vi "control_chart_axis.vi"(8 "stop":refnum<vi>, 9 "chart_array":refnum<vi>[](array[refnum]), 10 "chart_2":refnum<vi>, 11 "chart_1":refnum<vi>) -> ()   [LabVIEW 2019]
panel:
  in  "range_p1h":bool
  in  "range_p10m":bool
  in  "range_p5m":bool
  in  "chart_x_range":u32 caption="Time range"
  in  "auto_x_scale":bool caption="Time Scale"
  in  "auto_y_scale":bool caption="Vertical Scale"
  # "min"
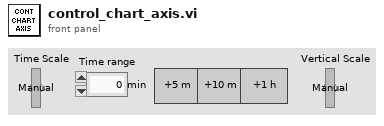
[diagram p1: front panel]
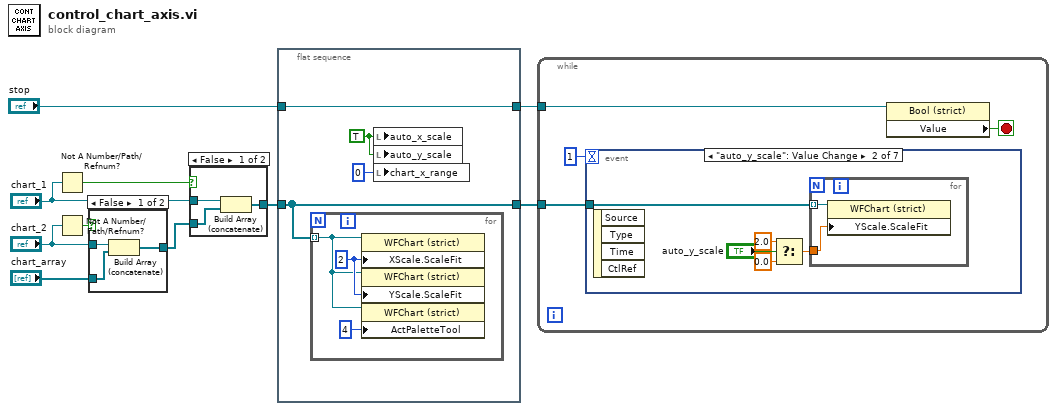
[diagram p0: block diagram]
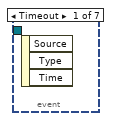
[diagram p4: hidden frame]
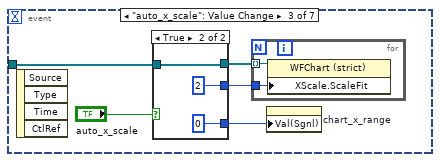
[diagram p5: hidden frame]
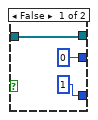
[diagram p6: hidden frame]
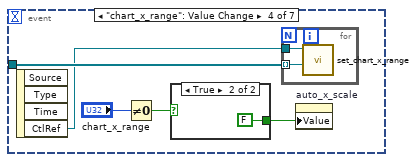
[diagram p7: hidden frame]
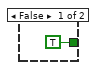
[diagram p8: hidden frame]
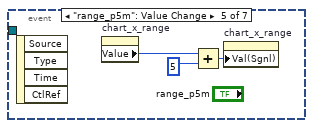
[diagram p9: hidden frame]
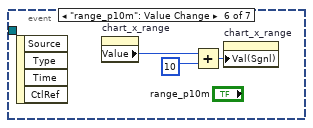
[diagram p10: hidden frame]
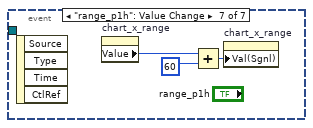
[diagram p11: hidden frame]
diagram:
  n1 = Not A Number/Path/Refnum?(number/path/refnum="chart_1") -> (NaN/Path/Refnum?=w7:bool)
  n2 = Not A Number/Path/Refnum?(number/path/refnum="chart_2") -> (NaN/Path/Refnum?=w4:bool)
  n3 = case shown="False" w4 {
    tunnel: "chart_array" -> [w12 w14]
    tunnel: "chart_2" -> [w13 _]
    tunnel: [w11 w14] -> w1
    frame False {
      n4 = Build Array (concatenate)(w13, w12) -> (w11:refnum<vi>[])
    }
    frame True {
    }
  }
  n5 = case shown="False" w7 {
    tunnel: "chart_1" -> [w16 _]
    tunnel: [w17 w18] -> w5
    tunnel: w1 -> [w15 w18]
    frame False {
      n6 = Build Array (concatenate)(w16, w15) -> (w17:refnum<vi>[])
    }
    frame True {
    }
  }
  n7 = flat-sequence {
    tunnel: w5 -> [w20]
    tunnel: [w20] -> w10
    tunnel: [w19] -> w9
    tunnel: "stop" -> [w19]
    frame #0 {
      w21 = TRUE ("auto_x_scale")
      n8 = for {
        tunnel: w20 -> [w24] mode=indexing
        w25 = u8 2 ("X Scale.Scale Fit")
        n9 = property class="WFChart (strict)"(reference=w24, "XScale.ScaleFit"=w25) -> ()  [unwired: 1 in, 2 out]
        n10 = property class="WFChart (strict)"(reference=w24, "YScale.ScaleFit"=w25) -> ()  [unwired: 1 in, 2 out]
        n11 = property class="WFChart (strict)"(reference=w24, "ActPaletteTool"=4 ("Palette:Active Tool")) -> ()  [unwired: 1 in, 2 out]
      }
      n12 = local write "auto_x_scale"(w21) -> ()
      n13 = local write "auto_y_scale"(w21) -> ()
      n14 = local write "chart_x_range"(u32 0 ("chart_x_range")) -> ()
    }
  }
  n15 = while {
    tunnel: w10 -> [w28]
    tunnel: w9 -> [w26]
    stop <- w27 stop-if-true
    n16 = event shown="[1] \"auto_y_scale\": Value Change" {
      selector: _ -> [_ _ _ _ _ _ _]
      dyn-events: _ -> [_ _ _ _ _ _ _]
      timeout: 1 -> [_ _ _ _ _ _ _]
      tunnel: w28 -> [_ w30 w38 w51 _ _ _]
      event Timeout {
        n17 = event-data() -> ()  [unwired: 1 in, 3 out]
      }
      event "auto_y_scale": Value Change {
        n18 = event-data() -> ()  [unwired: 1 in, 4 out]
        n19 = Select(t=2.0, s="auto_y_scale", f=0.0) -> (s? t:f=w33:dbl)
        n20 = for {
          tunnel: w33 -> [w36]
          tunnel: w30 -> [w35] mode=indexing
          n21 = property class="WFChart (strict)"(reference=w35, "YScale.ScaleFit"=w36) -> ()  [unwired: 1 in, 2 out]
        }
      }
      event "auto_x_scale": Value Change {
        n22 = event-data() -> ()  [unwired: 1 in, 4 out]
        n23 = case shown="True" "auto_x_scale" {
          tunnel: [1 ("chart_x_range") 0 ("chart_x_range")] -> w40
          tunnel: [u8 0 ("X Scale.Scale Fit") u8 2 ("X Scale.Scale Fit")] -> w39
          tunnel: w38 -> [w44 w47]
          tunnel: [w44 w47] -> w37
          frame False {
          }
          frame True {
          }
        }
        n24 = for {
          tunnel: w39 -> [w43]
          tunnel: w37 -> [w42] mode=indexing
          n25 = property class="WFChart (strict)"(reference=w42, "XScale.ScaleFit"=w43) -> ()  [unwired: 1 in, 2 out]
        }
        n26 = property on="chart_x_range" class="DigNum (strict)"("Val(Sgnl)"=w40) -> ()  [unwired: 2 in, 2 out]
      }
      event "chart_x_range": Value Change {
        n27 = event-data() -> ("CtlRef"=w50:refnum<vi>)  [unwired: 1 in, 3 out]
        n28 = Not Equal To 0?(x="chart_x_range") -> (x != 0?=w53:bool)
        n29 = case shown="True" w53 {
          tunnel: [TRUE ("auto_x_scale") FALSE ("auto_x_scale")] -> w52
          frame False {
          }
          frame True {
          }
        }
        n30 = for {
          tunnel: w51 -> [w56] mode=indexing
          tunnel: w50 -> [w55]
          n31 = call "set_chart_x_range.vi"("ref_chart"=w56, "ref_x_range"=w55) -> ()  [unwired: 10 in]
        }
        n32 = property on="auto_x_scale" class="Bool (strict)"("Value"=w52) -> ()  [unwired: 2 in, 2 out]
      }
      event "range_p5m": Value Change {
        n33 = event-data() -> ()  [unwired: 1 in, 4 out]
        n34 = property on="chart_x_range" class="DigNum (strict)"() -> ("Value"=w61:u32)  [unwired: 2 in, 2 out]
        n35 = Add(x=w61, y=5) -> (x+y=w60:u32)
        n36 = property on="chart_x_range" class="DigNum (strict)"("Val(Sgnl)"=w60) -> ()  [unwired: 2 in, 2 out]
      }
      event "range_p10m": Value Change {
        n37 = event-data() -> ()  [unwired: 1 in, 4 out]
        n38 = property on="chart_x_range" class="DigNum (strict)"() -> ("Value"=w64:u32)  [unwired: 2 in, 2 out]
        n39 = Add(x=w64, y=10) -> (x+y=w63:u32)
        n40 = property on="chart_x_range" class="DigNum (strict)"("Val(Sgnl)"=w63) -> ()  [unwired: 2 in, 2 out]
      }
      event "range_p1h": Value Change {
        n41 = event-data() -> ()  [unwired: 1 in, 4 out]
        n42 = property on="chart_x_range" class="DigNum (strict)"() -> ("Value"=w67:u32)  [unwired: 2 in, 2 out]
        n43 = Add(x=w67, y=60) -> (x+y=w66:u32)
        n44 = property on="chart_x_range" class="DigNum (strict)"("Val(Sgnl)"=w66) -> ()  [unwired: 2 in, 2 out]
      }
    }
    n45 = property class="Bool (strict)"(reference=w26) -> ("Value"=w27:bool)  [unwired: 1 in, 2 out]
  }
